vi "PH_HamamatsuCamera.evt call Set ROI.vi"(0 "i ref in":refnum<vi>, 2 "Instance":string, 3 "ROI":T1, 5 "error in (no error)":errorcluster) -> (14 "i ref out":refnum<vi>, 19 "error out":errorcluster)   [LabVIEW 2014, in "PH_HamamatsuCamera.lvlib"]
doc: "This VI sends a simple call for SetROI."
uses:
  PH_HamamatsuCamera.lvlib
  PH_HamamatsuCamera.ROI.ctl
  CSCore/CSSystem/CoreLib/CoreLib.int 2 byte array.vi
  CSCore/CSSystem/CoreLib/CoreLib.lvlib
  CSCore/BaseProcess/BaseProcess.lvlib
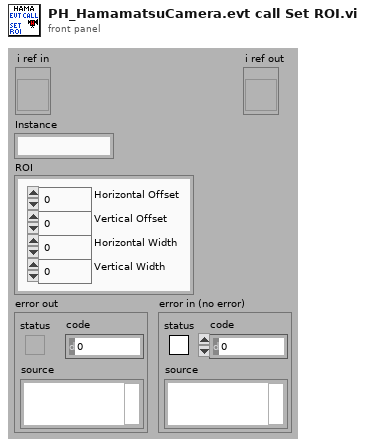
[diagram p1: front panel]
types:
  T1 = typedef "PH_HamamatsuCamera.lvlib/PH_HamamatsuCamera.ROI.ctl" = cluster{"Horizontal Offset":i32, "Vertical Offset":i32, "Horizontal Width":i32, "Vertical Width":i32}
  T2 = typedef "CoreDefs.rawDataType.ctl" = i8[]
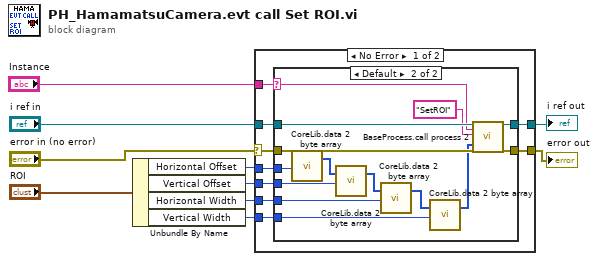
[diagram p0: block diagram]
diagram:
  n1 = Unbundle By Name("ROI") -> ("Horizontal Offset"=w3:i32, "Vertical Offset"=w2:i32, "Horizontal Width"=w4:i32, "Vertical Width"=w1:i32)
  n2 = case shown="No Error" "error in (no error)" {
    selector: "error in (no error)" -> [w16 w36]
    tunnel: [w19 w37] -> w8
    tunnel: [w18 w36] -> w7
    tunnel: "i ref in" -> [w17 w37]
    tunnel: "Instance" -> [w15 _]
    tunnel: w3 -> [w14 _]
    tunnel: w2 -> [w13 _]
    tunnel: w4 -> [w12 _]
    tunnel: w1 -> [w11 _]
    frame No Error {
      n3 = case shown="Default" w15 {
        selector: w15 -> [_ w22]
        tunnel: [w21 w35] -> w19
        tunnel: [w20 w34] -> w18
        tunnel: w17 -> [w21 w33]
        tunnel: w16 -> [w20 w31]
        tunnel: w14 -> [_ w30]
        tunnel: w13 -> [_ w29]
        tunnel: w12 -> [_ w27]
        tunnel: w11 -> [_ w25]
        frame "N/A" {
        }
        frame Default {
          n4 = call-poly "CoreLib.data 2 byte array.vi"("i32"=w30) -> ("byteArray out"=w28:T2)  [unwired: 18 in]
          n5 = call-poly "CoreLib.data 2 byte array.vi"("byteArray"=w28, "i32"=w29) -> ("byteArray out"=w26:T2)  [unwired: 17 in]
          n6 = call-poly "CoreLib.data 2 byte array.vi"("byteArray"=w26, "i32"=w27) -> ("byteArray out"=w24:T2)  [unwired: 17 in]
          n7 = call-poly "CoreLib.data 2 byte array.vi"("byteArray"=w24, "i32"=w25) -> ("byteArray out"=w23:T2)  [unwired: 17 in]
          n8 = call "BaseProcess.call process 2.vi"("i ref in"=w33, "Object"=w22, "Selector"="SetROI", "Data"=w23, "error in (no error)"=w31) -> ("i ref out"=w35:refnum<vi>, "error out"=w34:errorcluster)  [unwired: 13 in]
        }
      }
    }
    frame Error {
    }
  }
  "error out" <- w7
  "i ref out" <- w8
